vi "build config path.vi"(11 "Template in":refnum<class "Template.lvclass">) -> (0 "error out":errorcluster, 3 "Config Path":path)   [LabVIEW 2020, in "Template.lvlib" / "Template.lvclass"]
doc: "Builds the configuration file path\n\n%AppDir%\\configs\\<ActorName>_config.json"
uses:
  Template.lvclass
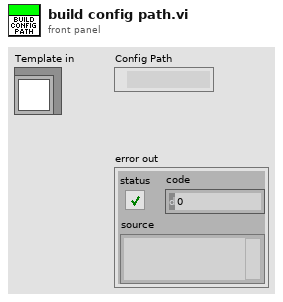
[diagram p1: front panel]
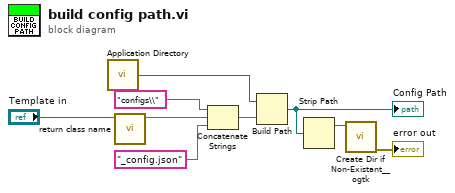
[diagram p0: block diagram]
diagram:
  n1 = call <vilib>:"Application Directory.vi"() -> ("Application Directory"=w1:path)
  n2 = call "return class name.vi"("Class in"="Template in") -> ("lowercase class name"=w3:string)  [unwired: 10 in]
  n3 = Concatenate Strings("configs\\" ("string"), w3, "_config.json" ("string")) -> (w5:string)
  n4 = Build Path(base path=w1, name or relative path=w5) -> (appended path=w9:path)
  "Config Path" <- w9
  n5 = Strip Path(path=w9) -> (stripped path=w8:path)  [unwired: 1 out]
  n6 = call <userlib>:"Create Dir if Non-Existant__ogtk.vi"("Directory Path"=w8) -> ("error out"=→"error out":errorcluster)  [unwired: 8 in, 2 out]
